vi "EE_ContactsQualityDisplay.vi"(0 "ChannelsDataNotifier in":T1, 5 "Contacts Quality Indicators":refnum<vi>[](array[refnum]), 11 "StopButton Refnum":refnum<vi>) -> (4 "ChannelsDataNotifier out":T1, 15 "error out":errorcluster)   [LabVIEW 2016, in "Emotiv Epoc.lvlib"]
uses:
  EE_Notifier_Refnum.ctl
  EE_Notifier_Data_Type.ctl
  EE_SignalStrength_enum.ctl
  EE_EEG_ContactQuality_enum.ctl
  Emotiv Epoc.lvlib
  EmotivEpocHeadsetControls.lvclass
panel:
  # "This VI is a part of BCI Design library, http://www.ru-bci.org \nCopyright © 2020, Sotnikov Peter, All rights reserved. License: CC BY-NC 4.0"
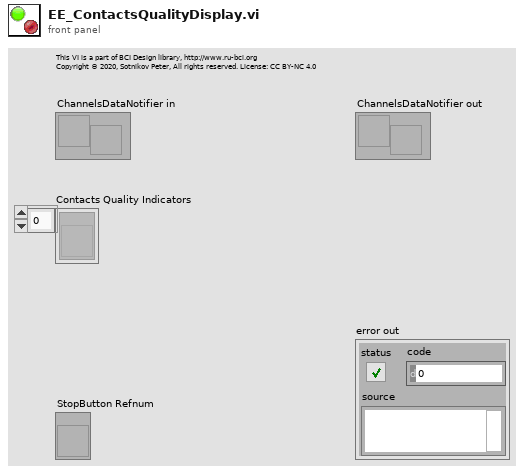
[diagram p1: front panel]
types:
  T1 = typedef "Emotiv Epoc.lvlib/EE_Notifier_Refnum.ctl" = refnum<notifier>
  T2 = typedef "Emotiv Epoc.lvlib/EE_EEG_ContactQuality_enum.ctl" = enum16{"EEG_CQ_NO_SIGNAL", "EEG_CQ_VERY_BAD", "EEG_CQ_POOR", "EEG_CQ_FAIR", "EEG_CQ_GOOD"}
  T3 = typedef "Emotiv Epoc.lvlib/EE_Notifier_Data_Type.ctl" = cluster{"EDK_Error":string, "Number of samples":u32, "Marker Waveform":waveform(dbl), "Array of EEG waveforms":waveform(dbl)[], "WirelessSignalStatus":T4, "EEG_ContactsQuality":T2[]}
  T4 = typedef "Emotiv Epoc.lvlib/EmotivEpocHeadsetControls.lvclass/EE_SignalStrength_enum.ctl" = enum32{"NO_SIGNAL", "BAD_SIGNAL", "GOOD_SIGNAL"}
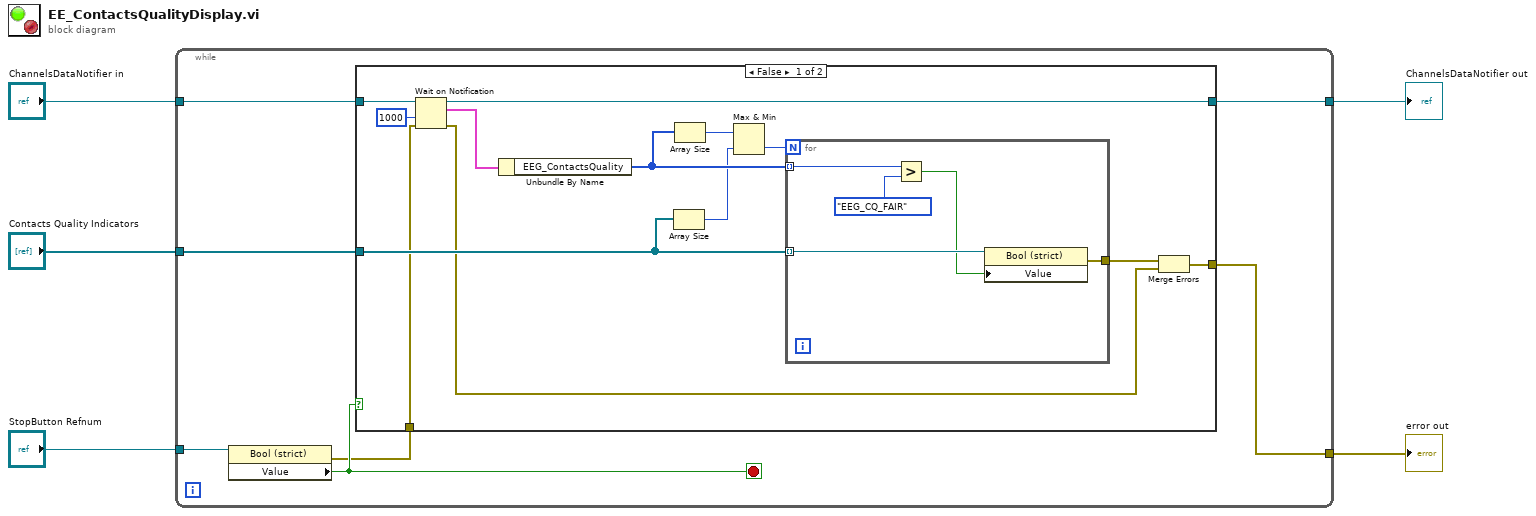
[diagram p0: block diagram]
diagram:
  n1 = while {
    tunnel: "StopButton Refnum" -> [w12]
    tunnel: [w11] -> w4
    tunnel: "ChannelsDataNotifier in" -> [w10]
    tunnel: [w9] -> w2
    tunnel: "Contacts Quality Indicators" -> [w8]
    stop <- w7 stop-if-true
    n2 = property class="Bool (strict)"(reference=w12) -> (error out=w6:errorcluster, "Value"=w7:bool)  [unwired: 1 in, 1 out]
    n3 = case shown="False" w7 {
      tunnel: [w25 w31] -> w11
      tunnel: w10 -> [w24 w32]
      tunnel: [w22 w32] -> w9
      tunnel: w8 -> [w20 _]
      tunnel: w6 -> [w14 w31]
      frame False {
        n4 = Wait on Notification(notifier=w24, timeout in ms (-1)=1000, error in (no error)=w14) -> (notifier out=w22:T1, notification=w21:T3, error out=w13:errorcluster)  [unwired: 1 in, 1 out]
        n5 = Unbundle By Name(w21) -> ("EEG_ContactsQuality"=w19:T2[])
        n6 = Array Size(array=w20) -> (size(s)=w17:i32)
        n7 = Array Size(array=w19) -> (size(s)=w18:i32)
        n8 = Max & Min(x=w18, y=w17) -> (min(x,y)=w16:i32)  [unwired: 1 out]
        n9 = for {
          N: w16 -> [_]
          tunnel: w19 -> [w29] mode=indexing
          tunnel: w20 -> [w30] mode=indexing
          tunnel: [w27] -> w15
          n10 = Greater?(x=w29, y=EE_EEG_ContactQuality_enum."EEG_CQ_FAIR") -> (0:w26:bool)
          n11 = property class="Bool (strict)"(reference=w30, "Value"=w26) -> (error out=w27:errorcluster)  [unwired: 1 in, 1 out]
        }
        n12 = Merge Errors(w15, w13) -> (w25:errorcluster)
      }
      frame True {
      }
    }
  }
  "error out" <- w4
  "ChannelsDataNotifier out" <- w2
